vi "FPGA.vi"() -> ()   [LabVIEW 2014]
uses:
  <vilib>/rvi/Emulation/niFpgaGetClockAttributes.vi
  <vilib>/rvi/Emulation/niFpgaSctlEmulationGetInTimedLoop.vi
  <vilib>/rvi/Emulation/niFpgaEmulationReportErrorSimple.vi
  <vilib>/rvi/eio/common/nirviEmuTemplateMethod_errors.vi
  <vilib>/rvi/interface/RandomDataEmulation/niFpgaRandomDataHandleErrors.vi
  <vilib>/rvi/Emulation/niFpgaCriticalErrorInLSC.vi
  <vilib>/eio/EIONode/EIONode.xnode
  <vilib>/rvi/DataTransferAndStorage/Container/XNode/niFpgaContainer.xnode
  <vilib>/rvi/interface/RandomDataEmulation/nirviRandomDataFpgaReadWriteTemplate.vi
panel:
  out "LED":bool
  in  "Iniciar\nmedicion":bool
  out "Periodo de muestreo":u32=26
  out "Timed Out?":bool
  out "Tick Count(mSec)":u32 caption="Tick Count(uSec)"
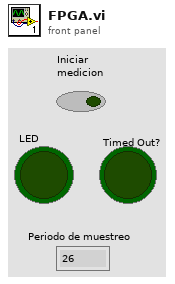
[diagram p1: front panel]
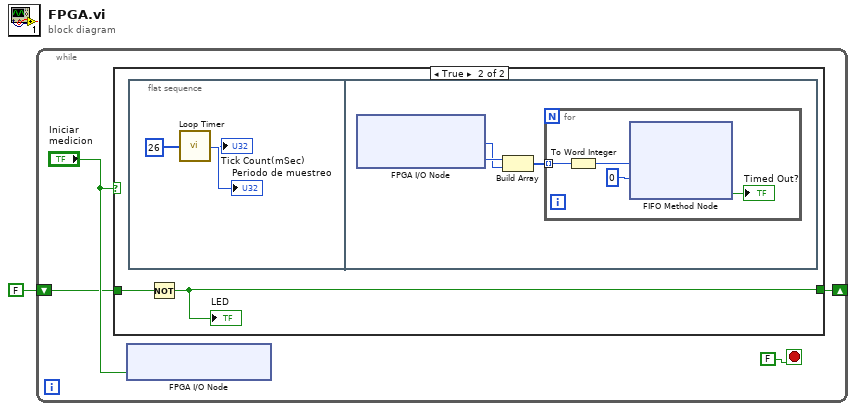
[diagram p0: block diagram]
diagram:
  n1 = while {
    shift-right: [w2] -> _
    shift-left: FALSE -> [w3]
    stop <- FALSE stop-if-true
    n2 = case shown="True" "Iniciar\nmedicion" {
      tunnel: [w6 w7] -> w2
      tunnel: w3 -> [w6 w8]
      frame False {
      }
      frame True {
        n3 = flat-sequence {
          frame #0 {
            w10 = u32 26 ("Sample Time")
            n4 = call "Loop Timer"("Count(uSec)"=w10) -> ("Tick Count(uSec)"=→"Tick Count(mSec)":u32)
            "Periodo de muestreo" <- w10
          }
          frame #1 {
            n5 = xnode "FPGA I/O Node"() -> ("ConnectorB/AI0"=w12:u16, "ConnectorB/AI1"=w13:u16)  [unwired: 2 in, 2 out]
            n6 = Build Array(w13, w12) -> (w11:u16[])
            n7 = for {
              tunnel: w11 -> [w17] mode=indexing
              n8 = To Word Integer(number=w17) -> (16bit integer=w16:i16)
              n9 = xnode ("FIFO Method Node")("Element"=w16, "Timeout"=0) -> ("Timed Out?"=→"Timed Out?":bool)  [unwired: 1 in, 1 out]
            }
          }
        }
        n10 = Not(x=w8) -> (.not. x?=w7:bool)
        "LED" <- w7
      }
    }
    n11 = xnode "FPGA I/O Node"("ConnectorA/DIO10"="Iniciar\nmedicion") -> ()  [unwired: 1 in, 1 out]
  }
